vi "Master on Desktop.vi"() -> ()   [LabVIEW 2019]
doc: "Demonstrates how to use Modbus functions to create a master communicating with a Modbus slave. It shows an interactive UI to allow users manually read and write the coils on the slave using TCP connection. Users can also change the timeout for reading operation if the network state is not good."
uses:
  <vilib>/Modbus/subvis/Modbus API/Modbus API.lvclass/Modbus API.ctl
  <vilib>/Modbus/subvis/Transmission Data Unit (ADU)/Transmission Data Unit/Transmission Data Unit.lvclass/Transmission Data Unit.ctl
  <vilib>/Modbus/master/Data Access/Read Timeout/Set Read Timeout.vi
  <vilib>/Modbus/subvis/Modbus API/Read Transmission Data Unit.vi
  <vilib>/Modbus/subvis/Modbus API/Write Transmission Data Unit.vi
  <vilib>/Modbus/subvis/Transmission Data Unit (ADU)/Transmission Data Unit/Data Access/timeouts/Write read operation timeout.vi
  <vilib>/Modbus/master/Modbus Master.lvclass
  C:/Program Files (x86)/National Instruments/LabVIEW 2019/vi.lib/Modbus/subvis/Modbus API/Modbus API.lvclass
  <vilib>/Modbus/master/Create Master Instance (TCP).vi
  <vilib>/Modbus/subvis/Transmission Data Unit (ADU)/Transmission Data Unit/Transmission Data Unit.lvclass
panel:
  in  "Set Read Timeout":bool
  in  "Read Timeout (ms)":i32=5000
  in  "Stop":bool
  in  "Read":bool
  out "Coil Values Read":u16
  in  "Write":bool
  in  "Coil Values to Write":u16
  # "Overview: Demonstrates the use of the Modbus Master VIs to create a Modbus master and use the Modbus master to read and write coil values on a Modbus slave.\nRequirements: LabVIEW Datalogging and Supervisory Control Module\nInstructions:\n1. Ensure Slave On Desktop.vi is already running.\n2. Run the VI.\n3. Click Stop to stop the VI."
  # "Write Operation"
  # "Read Operation"
  # "Set Timeout For Read Operation"
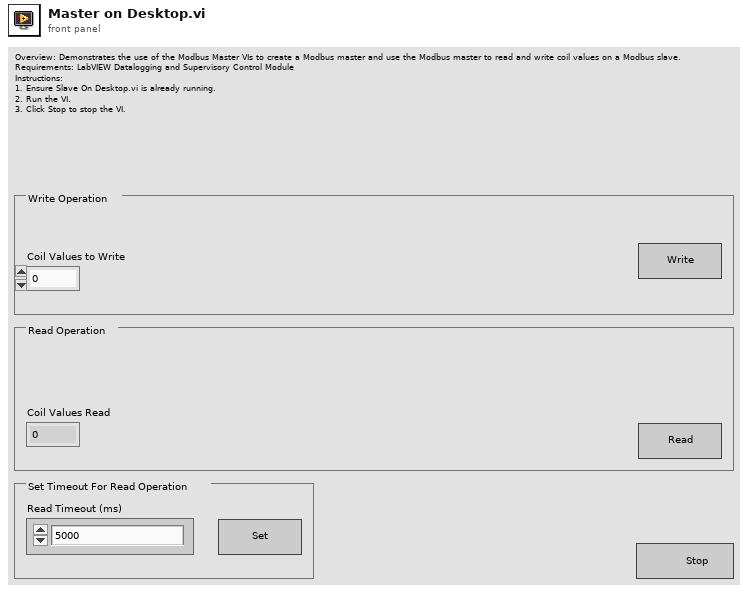
[diagram p1: front panel]
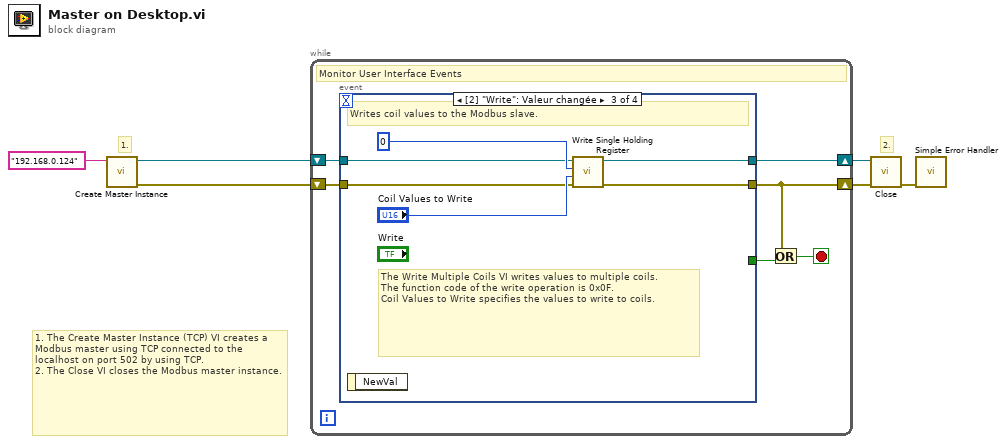
[diagram p0: block diagram]
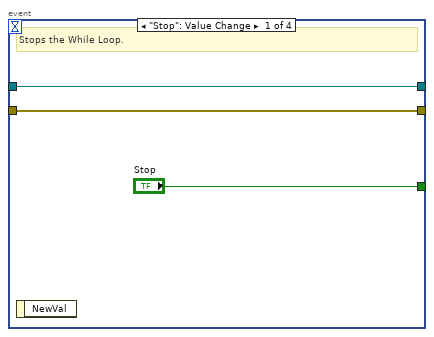
[diagram p2: hidden frame]
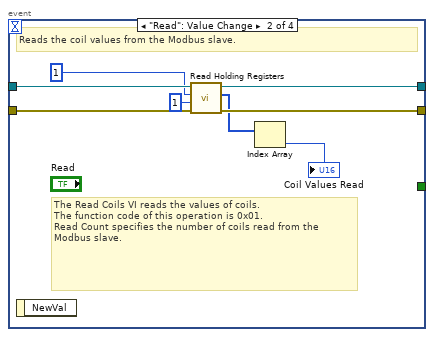
[diagram p3: hidden frame]
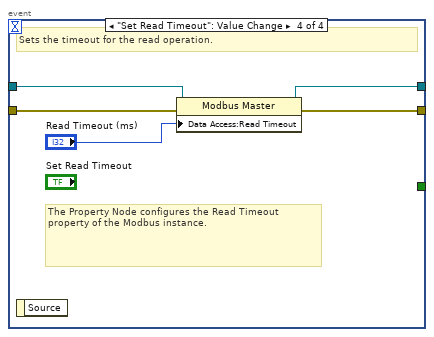
[diagram p4: hidden frame]
diagram:
  # "2."
  # "1."
  # "1. The Create Master Instance (TCP) VI creates a Modbus master using TCP connected to the localhost on port 502 by using TCP.\n2. The Close VI closes the Modbus master instance."
  n1 = call-poly <vilib>:"Create Master Instance.vi"("address"="192.168.0.124") -> ("error out"=w5:errorcluster, "TCP master instance"=w6:refnum<class "Modbus Master.lvclass">)  [unwired: 9 in]
  n2 = while {
    shift-right: [w11] -> w3
    shift-left: w6 -> [w12]
    shift-right: [w9] -> w4
    shift-left: w5 -> [w10]
    stop <- w7 stop-if-true
    # "Monitor User Interface Events"
    n3 = event shown="[2] \"Write\": Valeur changée" {
      selector: _ -> [_ _ _ _]
      dyn-events: _ -> [_ _ _ _]
      timeout: _ -> [_ _ _ _]
      tunnel: ["Stop" _ _ _] -> w8
      tunnel: w12 -> [w14 w23 w27 w34]
      tunnel: [w14 w22 w26 w32] -> w11
      tunnel: w10 -> [w15 w20 w25 w33]
      tunnel: [w15 w19 w24 w31] -> w9
      event "Stop": Value Change {
        # "Stops the While Loop."
        n4 = event-data() -> ()  [unwired: 1 in, 1 out]
      }
      event "Read": Value Change {
        # "The Read Coils VI reads the values of coils.\nThe function code of this operation is 0x01.\nRead Count specifies the number of coils read from the Modbus slave."
        # "Reads the coil values from the Modbus slave."
        n5 = event-data() -> ()  [unwired: 1 in, 1 out]
        n6 = call-dynamic "Read Holding Registers.vi"("error in (no error)"=w20, "number of holding registers"=u16 1, "starting address"=u16 1, "Modbus master in"=w23) -> ("error out"=w19:errorcluster, "register values"=w16:u16[], "Modbus master out"=w22:refnum<class "Modbus Master.lvclass">)  [unwired: 5 in]
        n7 = Index Array(array=w16) -> (element=→"Coil Values Read":u16)  [unwired: 1 in]
      }
      event "Write": Value Change {
        # "The Write Multiple Coils VI writes values to multiple coils.\nThe function code of the write operation is 0x0F.\nCoil Values to Write specifies the values to write to coils."
        # "Writes coil values to the Modbus slave."
        n8 = event-data() -> ()  [unwired: 1 in, 1 out]
        n9 = call-dynamic "Write Single Holding Register.vi"("error in (no error)"=w25, "holding register value"="Coil Values to Write", "address"=u16 0 ("starting address"), "Modbus master in"=w27) -> ("error out"=w24:errorcluster, "Modbus master out"=w26:refnum<class "Modbus Master.lvclass">)  [unwired: 6 in]
      }
      event "Set Read Timeout": Value Change {
        # "The Property Node configures the Read Timeout property of the Modbus instance."
        # "Sets the timeout for the read operation."
        n10 = event-data() -> ()  [unwired: 1 in, 1 out]
        n11 = property class="Modbus Master"(reference=w34, error in=w33, "Data Access:Read Timeout"="Read Timeout (ms)") -> (reference out=w32:refnum<class "Modbus Master.lvclass">, error out=w31:errorcluster)
      }
    }
    n12 = Or(x=w9, y=w8) -> (x .or. y?=w7:bool)
  }
  n13 = call-dynamic "Close.vi"("error in (no error)"=w4, "Modbus master in"=w3) -> ("error out"=w1:errorcluster)  [unwired: 9 in]
  n14 = call <vilib>:"Simple Error Handler.vi"("error in (no error)"=w1) -> ()  [unwired: 4 in, 5 out]
